vi "Msgbox - Message Handler.vi"(4 "Application (Default SRTRS)":string="SRTRS", 5 "Short Description (When DB Not Available)":string, 6 "Use DB":bool=TRUE, 7 "Description (When DB Not Available)":string, 8 "Error In (NA)":errorcluster, 9 "Post-Description":string, 10 "Pre-Description":string, 11 "<.?....> Message Code":string="<     >") -> (0 "MHandler Error":errorcluster, 2 "OK Out":bool, 3 "<. ....> + Pre-Description<PrePost>Post-Description":string)   [LabVIEW 2020]
uses:
  Variables/Global CMS.vi
  Variables/Global AMS.vi
  Variables/Global SRTRS.vi
panel:
  out "Q Error":errorcluster
  # "Test Codes\nComments\nNeed to set \nPlant, Language\nEnable INSERTS when testing"
  # "<I0101>Admin\n<E7105> Operator<PrePost>4070\n<E8107> Database Not Not Available  (en and zh)"
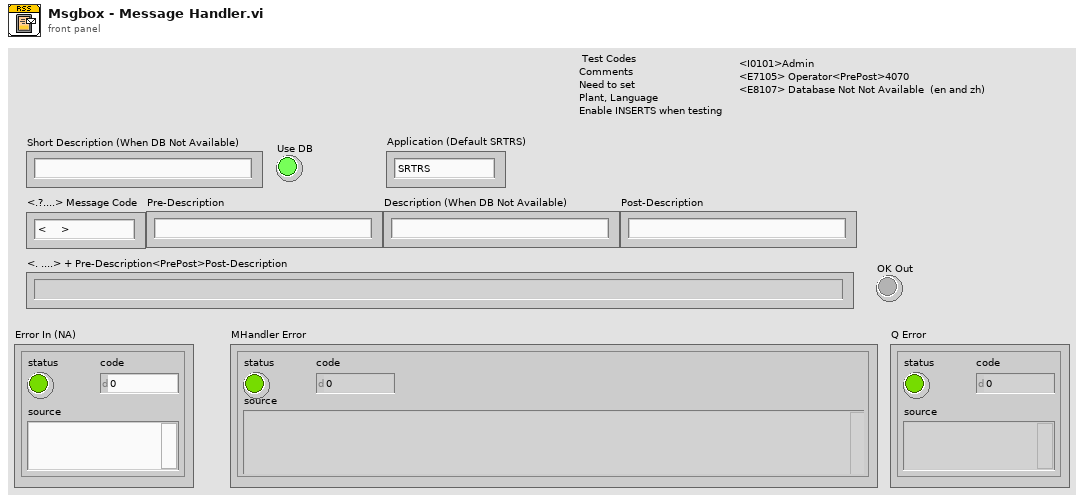
[diagram p1: front panel]
types:
  T1 = cluster{"Short Description (When DB Not Available)":string, "Description (When DB Not Available)":string}
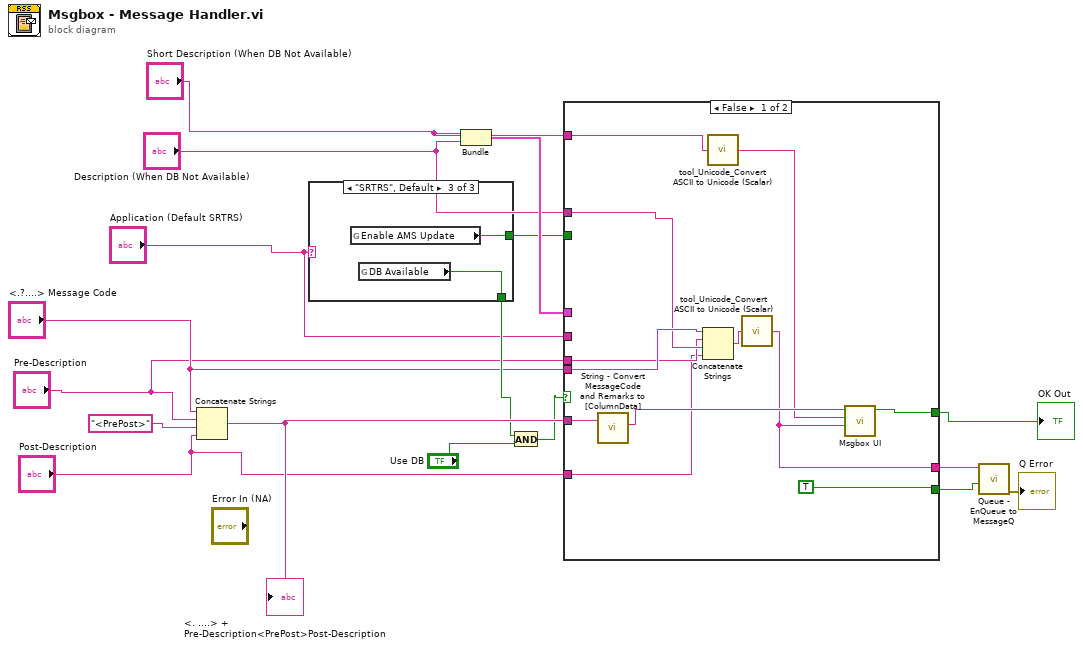
[diagram p0: block diagram]
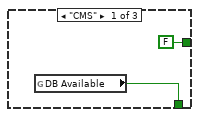
[diagram p2: hidden frame]
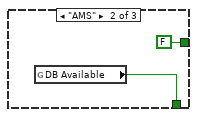
[diagram p3: hidden frame]
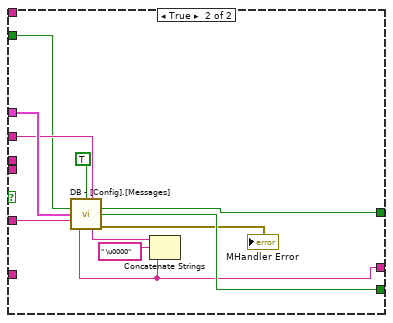
[diagram p4: hidden frame]
diagram:
  n1 = Concatenate Strings("<.?....> Message Code", "Pre-Description", "<PrePost>" ("string"), "Post-Description") -> (w16:string)
  "<. ....> + Pre-Description<PrePost>Post-Description" <- w16
  n2 = case shown="\"SRTRS\", Default" "Application (Default SRTRS)" {
    tunnel: [w19 w21 w23] -> w6
    tunnel: [FALSE ("Enable AMS Update") FALSE ("Enable AMS Update") w22] -> w3
    frame "CMS" {
      n3 = global read "Global CMS.vi" "DB Available"() -> (w19:bool)
    }
    frame "AMS" {
      n4 = global read "Global AMS.vi" "DB Available"() -> (w21:bool)
    }
    frame "SRTRS", Default {
      n5 = global read "Global SRTRS.vi" "Enable AMS Update"() -> (w22:bool)
      n6 = global read "Global SRTRS.vi" "DB Available"() -> (w23:bool)
    }
  }
  n7 = Bundle("Short Description (When DB Not Available)"="Short Description (When DB Not Available)", "Description (When DB Not Available)"="Description (When DB Not Available)") -> (w9:T1)  [unwired: 1 in]
  n8 = And(x=w6, y="Use DB") -> (x .and. y?=w11:bool)
  n9 = case shown="False" w11 {
    tunnel: w16 -> [w35 w46]
    tunnel: [w29 w39] -> w15
    tunnel: [TRUE w43] -> w14
    tunnel: [w34 w42] -> w13
    tunnel: w9 -> [_ w40]
    tunnel: "Description (When DB Not Available)" -> [w26 _]
    tunnel: "Short Description (When DB Not Available)" -> [w31 _]
    tunnel: "Application (Default SRTRS)" -> [_ w38]
    tunnel: "<.?....> Message Code" -> [w28 _]
    tunnel: w3 -> [_ w36]
    tunnel: "Pre-Description" -> [w25 _]
    tunnel: "Post-Description" -> [w24 _]
    frame False {
      n10 = call "String - Convert MessageCode and Remarks to [ColumnData].vi"("<. ....> + Pre-Description<PrePost>Post-Description"=w35) -> ("[MessageType]"=w33:string)  [unwired: 4 in, 6 out]
      n11 = Concatenate Strings(w28, w25, w26, w24) -> (w27:string)
      n12 = call "tool_Unicode_Convert ASCII to Unicode (Scalar).vi"("ASCII"=w31) -> ("Unicode"=w30:string)  [unwired: 4 in]
      n13 = call "tool_Unicode_Convert ASCII to Unicode (Scalar).vi"("ASCII"=w27) -> ("Unicode"=w29:string)  [unwired: 4 in]
      n14 = call "Msgbox UI.vi"("<xxxxxx> + Pre+Description+Post (Unicode)"=w29, "[ShortDescription] (Unicode)"=w30, "[MessageType]"=w33) -> ("OK Out"=w34:bool)  [unwired: 6 in, 2 out]
    }
    frame True {
      n15 = call "DB - [Config].[Messages].vi"("INSERT TO [SRTRS].[Execute].[MessageLog]"=TRUE ("INSERT TO [AMS].[Execute].[MessageLog]"), "Application (Default SRTRS)"=w38, "INSERT TO [AMS].[Execute].[MessageLog]"=w36, "Cluster (When DB Not Available)"=w40, "<.?...> + Pre-Description<PrePost>Post-Description"=w46) -> ("OK Out"=w42:bool, "<NoD>"=w43:bool, "[Remarks] Pre+Description+Post (Unicode)"=w39:string, "[ShortDescription] (Unicode)"=w45:string, "SUMMARY"=→"MHandler Error":errorcluster)  [unwired: 4 in, 2 out]
      n16 = Concatenate Strings(w45, " \u0000" ("string"), w39) -> ()  [unwired: 1 out]
    }
  }
  "OK Out" <- w13
  n17 = call "Queue - EnQueue to MessageQ.vi"("<NoD> Don't Display to UI"=w14, "Message"=w15) -> ("Error Out"=→"Q Error":errorcluster)  [unwired: 9 in]
